vi "Search Array by Controller Type.vi"(0 "Controller Array in":refnum<class "Controller Array.lvclass">, 1 "Controller Type":T1) -> (2 "Controller Array Out":refnum<class "Controller Array.lvclass">, 3 "Index of found":i32, 4 "Controller found":refnum<class "Generic Plugin.lvclass">)   [LabVIEW 2020, in "Controller Array.lvclass"]
doc: "Search the array of controllers for one of the same name. This VI will only return the first occurance. If no element was found, it returns an index of -1 and a generic controller object."
uses:
  Controller Array.lvclass
  Controller/Generic Plugin.lvclass
  Controller/Controller Type.ctl
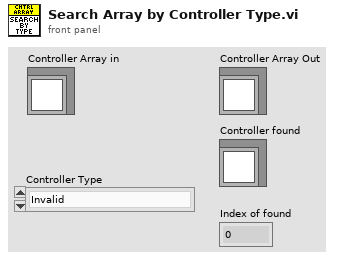
[diagram p1: front panel]
types:
  T1 = typedef "Generic Plugin.lvclass/Controller Type.ctl" = enum16{"Invalid", "Temperature Controller", "Pump Controller", "Generic Optimizer", "LC Parser"}
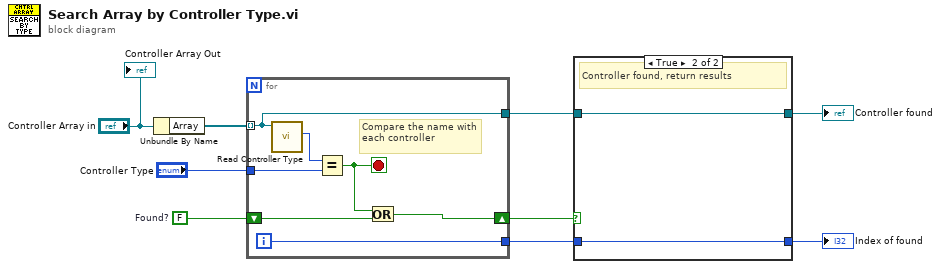
[diagram p0: block diagram]
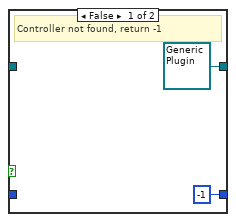
[diagram p2: hidden frame]
diagram:
  w7 = FALSE  # Found?
  n1 = Unbundle By Name("Controller Array in") -> ("Array"=w9:refnum<class "Generic Plugin.lvclass">[])
  n2 = for {
    tunnel: w9 -> [w14] mode=indexing
    tunnel: "Controller Type" -> [w15]
    tunnel: [w14] -> w3
    tunnel: [w13] -> w5
    shift-right: [w11] -> w6
    shift-left: w7 -> [w12]
    i -> [w13]
    stop <- w10 stop-if-true
    # "Compare the name with each controller"
    n3 = call "Read Controller Type.vi"("Generic Controller in"=w14) -> ("Controller Type"=w16:T1)  [unwired: 8 in, 2 out]
    n4 = Equal?(x=w16, y=w15) -> (x = y?=w10:bool)
    n5 = Or(x=w10, y=w12) -> (x .or. y?=w11:bool)
  }
  n6 = case shown="True" w6 {
    tunnel: [-1 w20] -> w4
    tunnel: w5 -> [_ w20]
    tunnel: w3 -> [_ w19]
    tunnel: [refnum<class "Generic Plugin.lvclass"> refnum ("Controller.lvclass") w19] -> w2
    frame False {
      # "Controller not found, return -1"
    }
    frame True {
      # "Controller found, return results"
    }
  }
  "Index of found" <- w4
  "Controller found" <- w2
  "Controller Array Out" <- "Controller Array in"
